vi "Find All Items with Property.vi"(8 "error in":errorcluster, 10 "Property Name":string, 11 "Section Ref in":T1 format="%.0x") -> (0 "error out":errorcluster, 2 "Item Refs":T1[](array[typedef]) format="%.0x", 3 "Section Ref out":T1 format="%.0x", 4 "Found":bool)   [LabVIEW 2020, in "Routing and Faulting Hardware API.lvlib"]
doc: "Derived from \"NI VeriStand - Search for All Items by Property.vi\", but ignores errors on getting properties and checks for property existence instead of a specific property value."
uses:
  Routing and Faulting Hardware API.lvlib
  <vilib>/NI VeriStand/Custom Device API/Custom Device Item Ref.ctl
  NationalInstruments.VeriStand.SystemDefinitionAPI
  NationalInstruments.VeriStand.SystemStorage
  <vilib>/NI VeriStand/Custom Device API/Custom Device API.lvlib
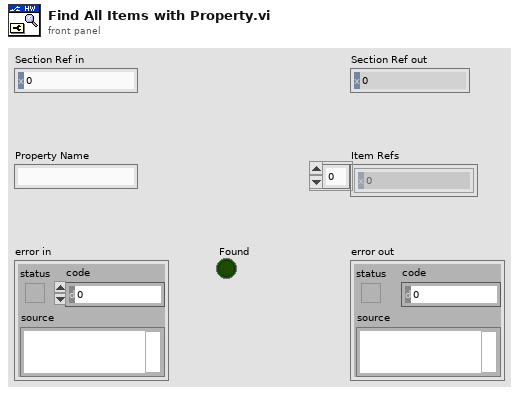
[diagram p1: front panel]
types:
  T1 = typedef "Custom Device API.lvlib/Custom Device Item Ref.ctl" = u64
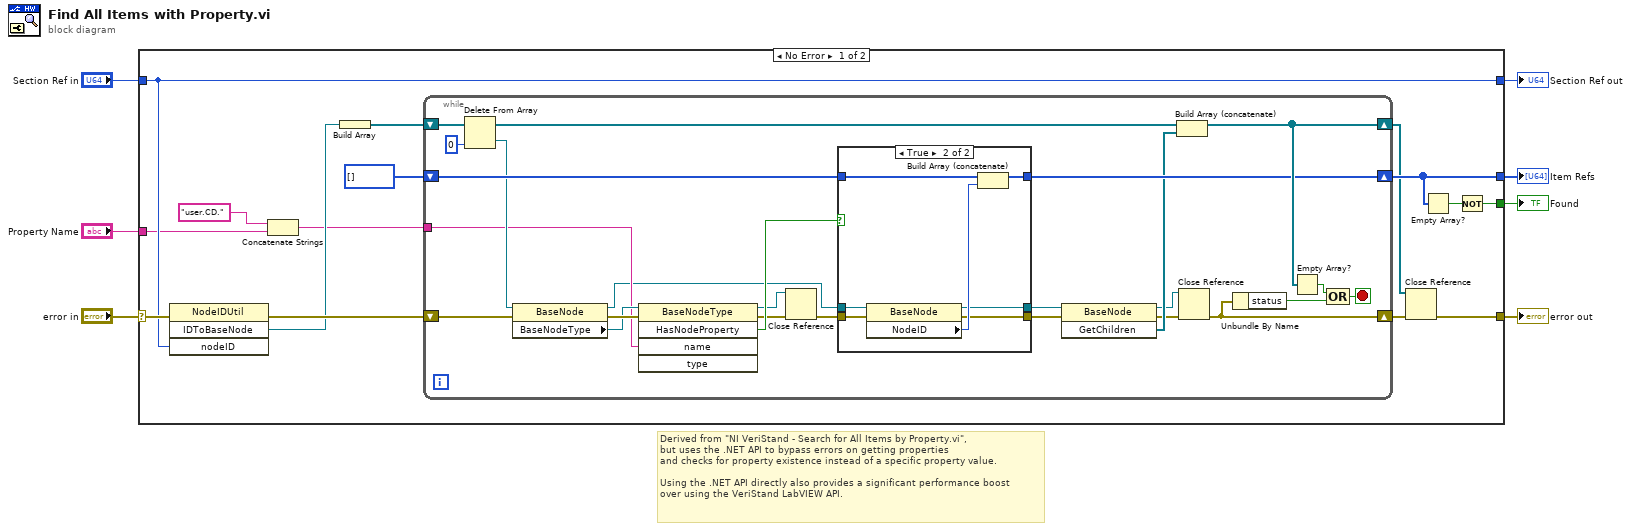
[diagram p0: block diagram]
diagram:
  # "Derived from \"NI VeriStand - Search for All Items by Property.vi\",\nbut uses the .NET API to bypass errors on getting properties\nand checks for property existence instead of a specific property value.\n\nUsing the .NET API directly also provides a significant performance boost\nover using the VeriStand LabVIEW API."
  n1 = case shown="No Error" "error in" {
    selector: "error in" -> [w17 w59]
    tunnel: "Section Ref in" -> [w15 w58]
    tunnel: "Property Name" -> [w12 _]
    tunnel: [w9 w59] -> w5
    tunnel: [w20 _] -> w4
    tunnel: [w18 _] -> w3
    tunnel: [w15 w58] -> w1
    frame No Error {
      n2 = invoke class="NodeIDUtil" method="IDToBaseNode"(error in=w17, "nodeID"=w15) -> (error out=w16:errorcluster, "IDToBaseNode"=w14:refnum<k24>)  [unwired: 2 in, 2 out]
      n3 = Concatenate Strings("user.CD." ("string"), w12) -> (w11:string)
      n4 = Build Array(w14) -> (w22:refnum<k24>[])
      n5 = while {
        shift-right: [w29] -> w10
        shift-left: w16 -> [w38]
        shift-right: [w44] -> w8
        shift-left: w22 -> [w47]
        tunnel: w11 -> [w34]
        shift-right: [w39] -> w20
        shift-left: T1[] [] ("appended array") -> [w40]
        stop <- w41 stop-if-true
        n6 = Delete From Array(array=w47, index=0) -> (deleted portion=w37:refnum<k24>, array with subset deleted=w45:refnum<k24>[])  [unwired: 1 in]
        n7 = property class="BaseNode"(reference=w37, error in=w38) -> (reference out=w32:refnum<k24>, error out=w36:errorcluster, "BaseNodeType"=w35:refnum<k24>)
        n8 = invoke class="BaseNodeType" method="HasNodeProperty"(reference=w35, error in=w36, "name"=w34) -> (reference out=w26:refnum<k24>, error out=w27:errorcluster, "HasNodeProperty"=w33:bool)  [unwired: 2 in, 2 out]
        n9 = Close Reference(reference=w26, error in (no error)=w27) -> (error out=w25:errorcluster)
        n10 = case shown="True" w33 {
          tunnel: w40 -> [w50 w57]
          tunnel: [w50 w56] -> w39
          tunnel: w32 -> [w48 w55]
          tunnel: w25 -> [w49 w53]
          tunnel: [w49 w52] -> w24
          tunnel: [w48 w51] -> w23
          frame False {
          }
          frame True {
            n11 = property class="BaseNode"(reference=w55, error in=w53) -> (reference out=w51:refnum<k24>, error out=w52:errorcluster, "NodeID"=w54:u64)
            n12 = Build Array (concatenate)(w57, w54) -> (w56:T1[])
          }
        }
        n13 = invoke class="BaseNode" method="GetChildren"(reference=w23, error in=w24) -> (reference out=w28:refnum<k24>, error out=w30:errorcluster, "GetChildren"=w31:refnum<k24>[])  [unwired: 1 in]
        n14 = Build Array (concatenate)(w45, w31) -> (w44:refnum<k24>[])
        n15 = Close Reference(reference=w28, error in (no error)=w30) -> (error out=w29:errorcluster)
        n16 = Unbundle By Name(w29) -> ("status"=w43:bool)
        n17 = Empty Array?(array=w44) -> (empty?=w42:bool)
        n18 = Compound Arithmetic op=OR(w42, w43) -> (w41:bool)
      }
      n19 = Close Reference(reference=w8, error in (no error)=w10) -> (error out=w9:errorcluster)
      n20 = Empty Array?(array=w20) -> (empty?=w19:bool)
      n21 = Not(x=w19) -> (.not. x?=w18:bool)
    }
    frame Error {
    }
  }
  "Found" <- w3
  "error out" <- w5
  "Section Ref out" <- w1
  "Item Refs" <- w4
